vi "Detect Shapes.vi"() -> ()   [LabVIEW 2020, in "examples.lvlib"]
doc: "Demonstrate Thresholding, Finding Contours and Using Approximate Poly to Identify simple shapes."
uses:
  examples.lvlib
  feature_detection/Contour Retrieval Modes.ctl
  feature_detection/Contour Approximation Mode.ctl
  image/ARGB Colour.ctl
  image/New Image (ARGB Preallocated).vi
  image/Copy Pixmap to Image (ARGB Flatten Mask).vi
  image/Draw Image to Picture (ARGB).vi
  image/Threshold (Binary).vi
  image/Draw Image to Picture (Greyscale).vi
  shape/Approximate Polygon (Douglas-Peucker).vi
  image/Draw Filled Poly (ARGB).vi
  image/New Image (ARGB Preallocated).vi/3321fa97-f432-4e1e-8db9-a0df79aed21b.vi
  image/ARGB Colour to U32 Pixel Value.vi
  image/Copy Pixmap to Image (ARGB Flatten Mask).vi/7d03ccf7-b889-4e8d-9f2a-57831e73dbde.vi
  image/Draw Image to Picture (ARGB).vi/8cd07b1b-062e-4fe4-9e87-2eb3dc89fe0e.vi
  image/New Image (Greyscale Preallocated).vi/6598b9e0-8a08-46f5-91fd-ca1b87217137.vi
  image/ARGBExtractChannel.vi
  image/ThresholdCore.vi
  image/Draw Image to Picture (Greyscale).vi/9ae995ca-ccda-485c-89ac-02736fde3e8e.vi
  image/Draw Filled Poly (ARGB).vi/e24a04ad-8575-4d64-b8af-da4c51ecb9cd.vi
  image/FixPixmap.vi
  image/Default8bitColourMap.vi
  <vilib>/Utility/error.llb/Error Cluster From Error Code.vi
  image/image.lvlib
  feature_detection/feature_detection.lvlib
  shape/shape.lvlib
panel:
  out "Input":picture
  out "Thresholded":picture
  out "Draw Contours On Original Image":picture
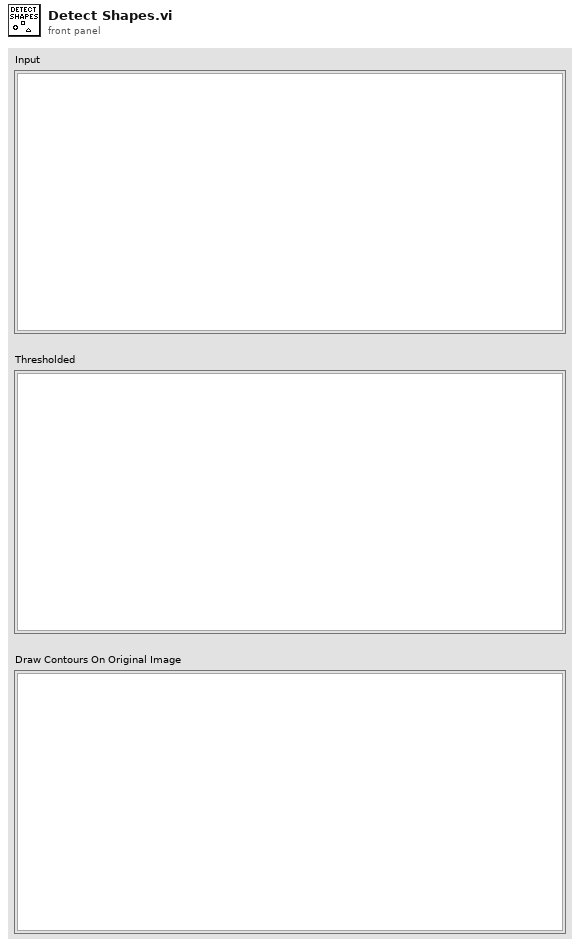
[diagram p1: front panel]
types:
  T1 = typedef "feature_detection.lvlib/Contour Approximation Mode.ctl" = enum16{"NONE", "SIMPLE", "TC89_L1", "TC89_KCOS"}
  T2 = typedef "feature_detection.lvlib/Contour Retrieval Modes.ctl" = enum16{"EXTERNAL", "LIST", "CCOMP", "TREE"}
  T3 = typedef "imagedata.ctl" = cluster{"image type":i32, "image depth":i32, "image":u8[], "mask":u8[], "colors":u32[], "Rectangle":cluster{"left":i16, "top":i16, "right":i16, "bottom":i16}}
  T4 = typedef "image.lvlib/ARGB Image.ctl" = refnum<data-value>
  T5 = typedef "image.lvlib/Greyscale Image.ctl" = refnum<data-value>
  T6 = typedef "feature_detection.lvlib/Found Contour.ctl" = cluster{"Points":T7[], "Hierarchy":T8}
  T7 = typedef "common.lvlib/Image Point (Integer).ctl" = cluster{"x":i32, "y":i32}
  T8 = typedef "feature_detection.lvlib/Contour Hierarchy.ctl" = cluster{"Next Contour Index":i32, "Previous Contour Index":i32, "First Child Contour Index":i32, "Parent Contour Index":i32}
  T9 = typedef "image.lvlib/ARGB Colour.ctl" = cluster{"Alpha":u8, "RGB":u32}
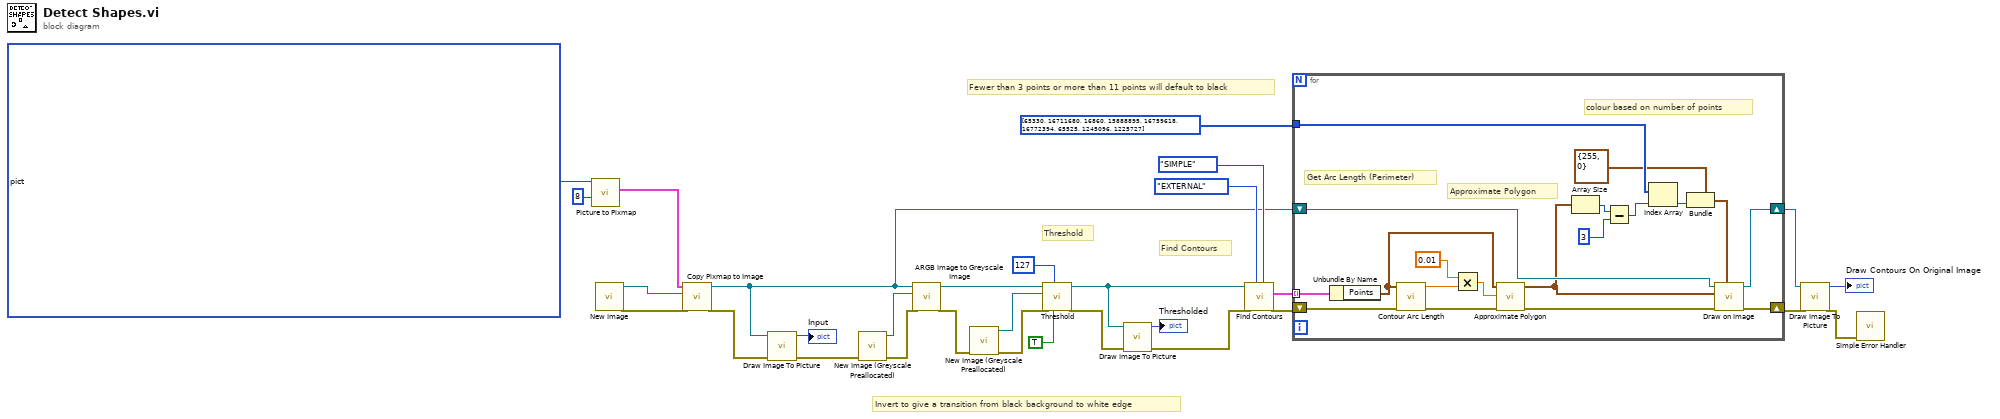
[diagram p0: block diagram]
diagram:
  # "Invert to give a transition from black background to white edge"
  # "Find Contours"
  # "Threshold"
  # "Fewer than 3 points or more than 11 points will default to black"
  n1 = call <vilib>:"Picture to Pixmap.vi"("depth"=8, "picture"=picture bytes[442122] ("Input 2")) -> ("image data"=w1:T3)  [unwired: 8 in, 1 out]
  n2 = call-poly "New Image.vi"() -> ("error out"=w29:errorcluster, "ARGB Image"=w30:T4)  [unwired: 10 in]
  n3 = call-poly "Copy Pixmap to Image.vi"("error in (no error)"=w29, "ARGB Image Destination in"=w30, "Pixmap Image Data"=w1) -> ("error out"=w10:errorcluster, "ARGB Image Destination"=w11:T4)  [unwired: 7 in]
  n4 = call-poly "Draw Image To Picture.vi"("error in (no error)"=w10, "ARGB Image Source in"=w11) -> ("error out"=w9:errorcluster, "Picture"=→"Input":picture)  [unwired: 8 in]
  n5 = call "New Image (Greyscale Preallocated).vi"("error in (no error)"=w9) -> ("error out"=w18:errorcluster, "Greyscale Image"=w17:T5)  [unwired: 9 in]
  n6 = call "ARGB Image to Greyscale Image.vi"("error in (no error)"=w18, "Greyscale Image Destination in"=w17, "ARGB Image Source in"=w11) -> ("error out"=w16:errorcluster, "Greyscale Image Destination"=w15:T5)  [unwired: 7 in]
  n7 = call "New Image (Greyscale Preallocated).vi"("error in (no error)"=w16) -> ("error out"=w27:errorcluster, "Greyscale Image"=w28:T5)  [unwired: 9 in]
  n8 = call-poly "Threshold.vi"("Invert? (Default: False)"=TRUE, "Threshold"=u8 127, "error in (no error)"=w27, "Threshold Result in"=w28, "Greyscale Image-Source in"=w15) -> ("error out"=w8:errorcluster, "Threshold Result"=w6:T5)  [unwired: 5 in]
  n9 = call-poly "Draw Image To Picture.vi"("error in (no error)"=w8, "Greyscale Image Source in"=w6) -> ("error out"=w7:errorcluster, "Picture"=→"Thresholded":picture)  [unwired: 8 in]
  n10 = call "Find Contours.vi"("Contour Approximation Mode (Default: SIMPLE)"=Contour_Approximation_Mode."SIMPLE", "Contour Retrieval Modes (Default: TREE)"=Contour_Retrieval_Modes."EXTERNAL", "error in (no error)"=w7, "Greyscale Image in"=w6) -> ("error out"=w20:errorcluster, "Found Contours"=w19:T6[])  [unwired: 5 in, 1 out]
  n11 = for {
    shift-right: [w48] -> w23
    shift-left: w20 -> [w49]
    tunnel: w19 -> [w44] mode=indexing
    shift-right: [w40] -> w13
    shift-left: w11 -> [w41]
    tunnel: u32[] [65330, 16711680, 16860, 15888895, 16759618, 16772394, 65525, 1245096, 1225727] -> [w37]
    # "Approximate Polygon"
    # "Get Arc Length (Perimeter)"
    # "colour based on number of points"
    n12 = Unbundle By Name(w44) -> ("Points"=w46:T7[])
    n13 = call "Contour Arc Length.vi"("error in (no error)"=w49, "Points in"=w46) -> ("error out"=w43:errorcluster, "Arc Length"=w45:dbl)  [unwired: 8 in]
    n14 = Multiply(x=0.01, y=w45) -> (x*y=w31:dbl)
    n15 = call-poly "Approximate Polygon.vi"("error in (no error)"=w43, "Epsilon"=w31, "Points in"=w46) -> ("error out"=w47:errorcluster, "Points out"=w39:T7[])  [unwired: 7 in]
    n16 = Array Size(array=w39) -> (size(s)=w38:i32)
    n17 = Subtract(x=w38, y=3) -> (x-y=w33:i32)
    n18 = Index Array(array=w37, index=w33) -> (element=w34:u32)
    n19 = Bundle(cluster=T9 {"Alpha"=255, "RGB"=0} ("ARGB Colour"), "RGB"=w34) -> (w35:T9)  [unwired: 1 in]
    n20 = call-poly "Draw on Image.vi"("ARGB Colour"=w35, "error in (no error)"=w47, "Points"=w39, "ARGB Image in"=w41) -> ("error out"=w48:errorcluster, "ARGB Image"=w40:T4)  [unwired: 6 in]
  }
  n21 = call-poly "Draw Image To Picture.vi"("error in (no error)"=w23, "ARGB Image Source in"=w13) -> ("error out"=w12:errorcluster, "Picture"=→"Draw Contours On Original Image":picture)  [unwired: 8 in]
  n22 = call <vilib>:"Simple Error Handler.vi"("error in (no error)"=w12) -> ()  [unwired: 4 in, 5 out]
